vi "Server.vi"() -> ()   [LabVIEW 2019]
doc: "The myRIO Project template acquires acceleration data from the onboard accelerometer and displays the changes of acceleration values in a waveform chart."
uses:
  <vilib>/myRIO/Common/Instrument Driver Framework/myRIO v1.0/UART/vis/myRIO v1.0 Close UART.vi
  <vilib>/myRIO/Common/Instrument Driver Framework/Utilities/vis/FPGA Ref Manager.vi
  <vilib>/myRIO/Common/Instrument Driver Framework/myRIO v1.0/myRIO v1.0 Reset FPGA.vi
  <vilib>/myRIO/Common/Instrument Driver Framework/myRIO v1.0/IRQ/vis/myRIO v1.0 IRQ Info FGV.vi
  <vilib>/myRIO/Common/Instrument Driver Framework/myRIO v1.0/IRQ/vis/myRIO v1.0 Timer IRQ Info FGV.vi
  <vilib>/myRIO/Common/Instrument Driver Framework/myRIO v1.0/IRQ/vis/myRIO v1.0 ISR Agent.vi
  <vilib>/myRIO/Instrument Drivers/Utilities/vis/Reset Index.vi
  <vilib>/myRIO/Common/Instrument Driver Framework/myRIO v1.0/Resource Manager/vis/myRIO v1.0 Block Write Resource Manager.vi
  <vilib>/myRIO/Instrument Drivers/Utilities/Utilities.lvlib
panel:
  out "Waveform Chart 2":dbl(graph)
  out "Waveform Chart":dbl(graph)
  in  "Client Closed 2":string="The client VI closed the connection."
  out "OUT 2":dbl
  out "OUT":dbl
  in  "Boolean":bool
  out "output array 2":dbl[](array[numeric])
  in  "Ki 4":dbl(slide) scale=0.001..0.1
  in  "Kd 4":dbl(slide) scale=0.01..0.5
  in  "Kp 4":dbl(slide)=2.0 scale=1.0..5.0
  out "output array":dbl[](array[numeric])
  in  "Ki 3":dbl(slide) scale=0.001..0.1
  in  "Kd 3":dbl(slide) scale=0.01..0.5
  in  "Kp 3":dbl(slide)=2.0 scale=1.0..5.0
  in  "Ki 2":dbl(slide) scale=0.01..1.0
  in  "Kd 2":dbl(slide)=0.1 scale=0.001..1.0
  in  "Kp 2":dbl(slide)=3.0 scale=0.5..3.0
  in  "PWM freq [Hz] 2":dbl(slide)=250.0 scale=40.0..1000.0
  in  "Fi 2":dbl(slide) scale=-0.4..0.4
  in  "Reset Counter 2":bool
  in  "Ki 1":dbl(slide) scale=0.01..1.0
  in  "Kd 1":dbl(slide)=0.1 scale=0.001..1.0
  in  "Stop":bool
  in  "Kp 1":dbl(slide)=3.0 scale=0.5..3.0
  in  "PWM freq [Hz] 1":dbl(slide)=250.0 scale=40.0..1000.0
  in  "Fi 1":dbl(slide) scale=-0.4..0.4
  in  "Reset Counter 1":bool
  in  "Client Closed":string="The client VI closed the connection."
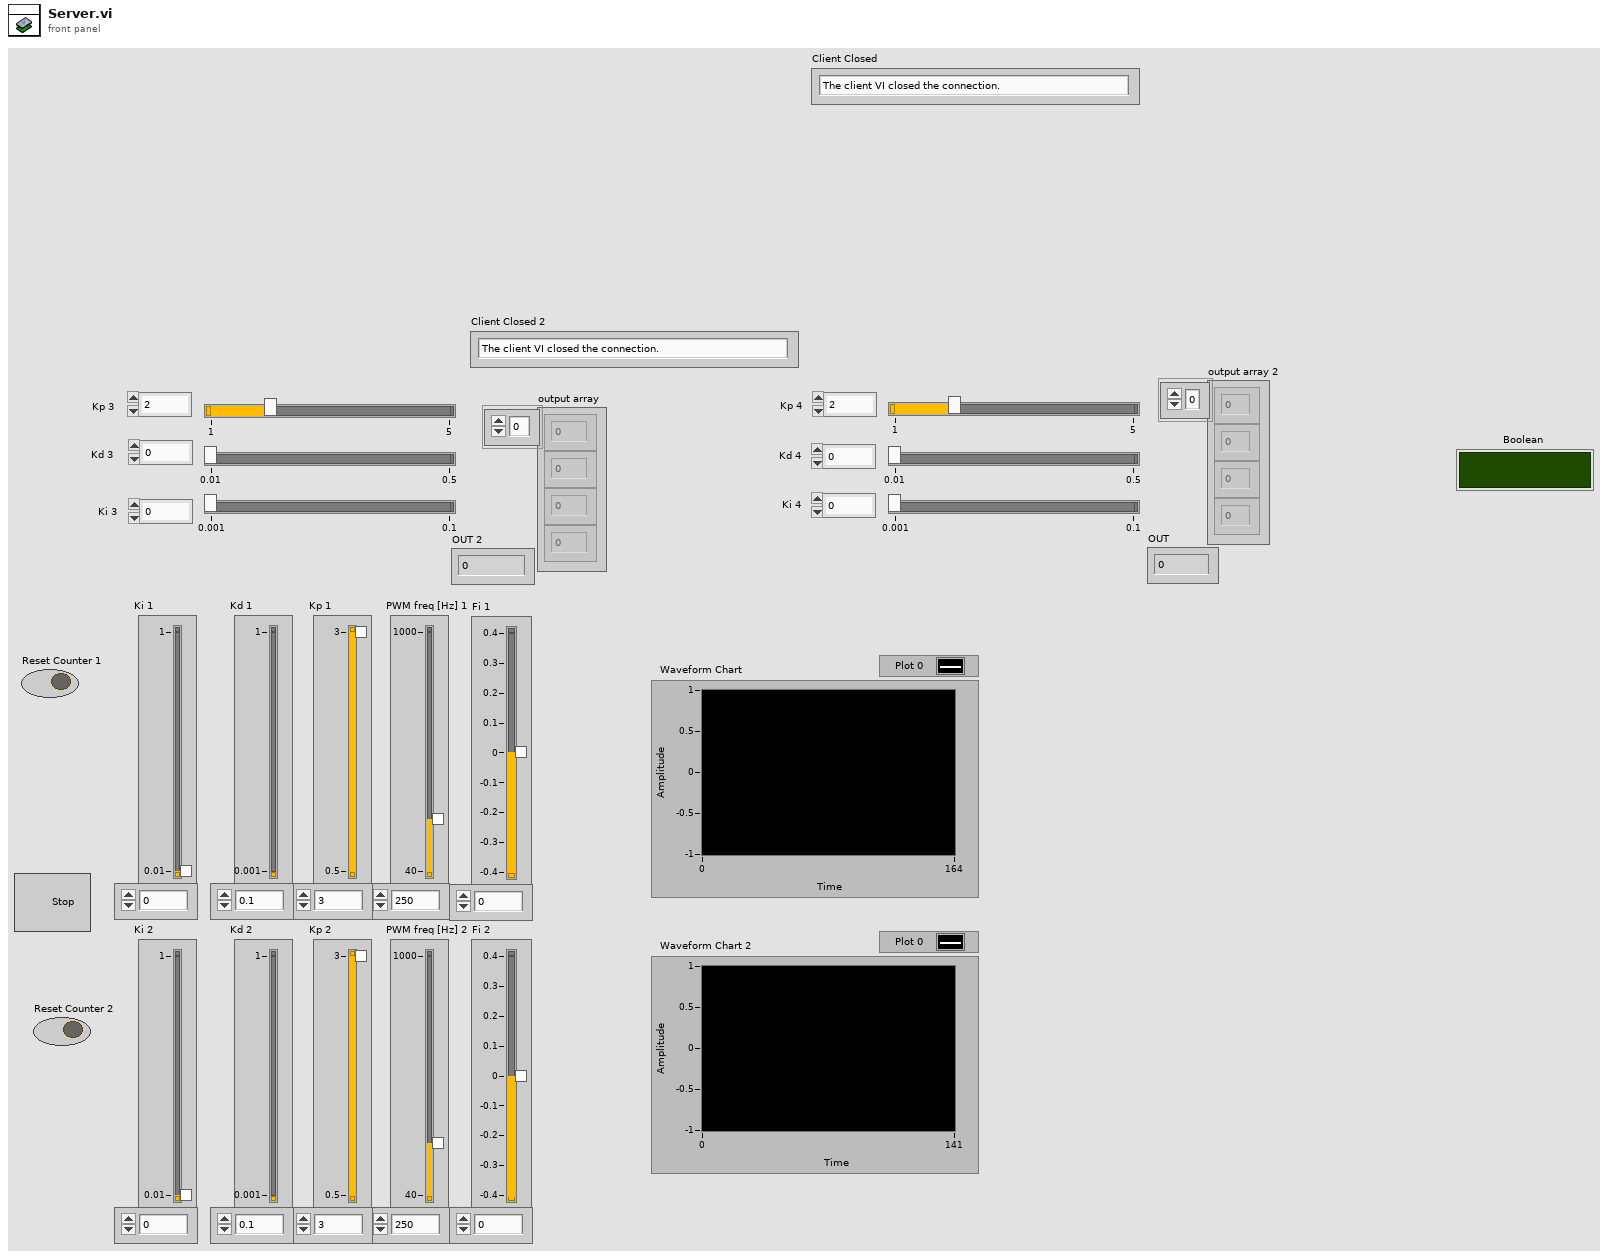
[diagram p1: front panel]
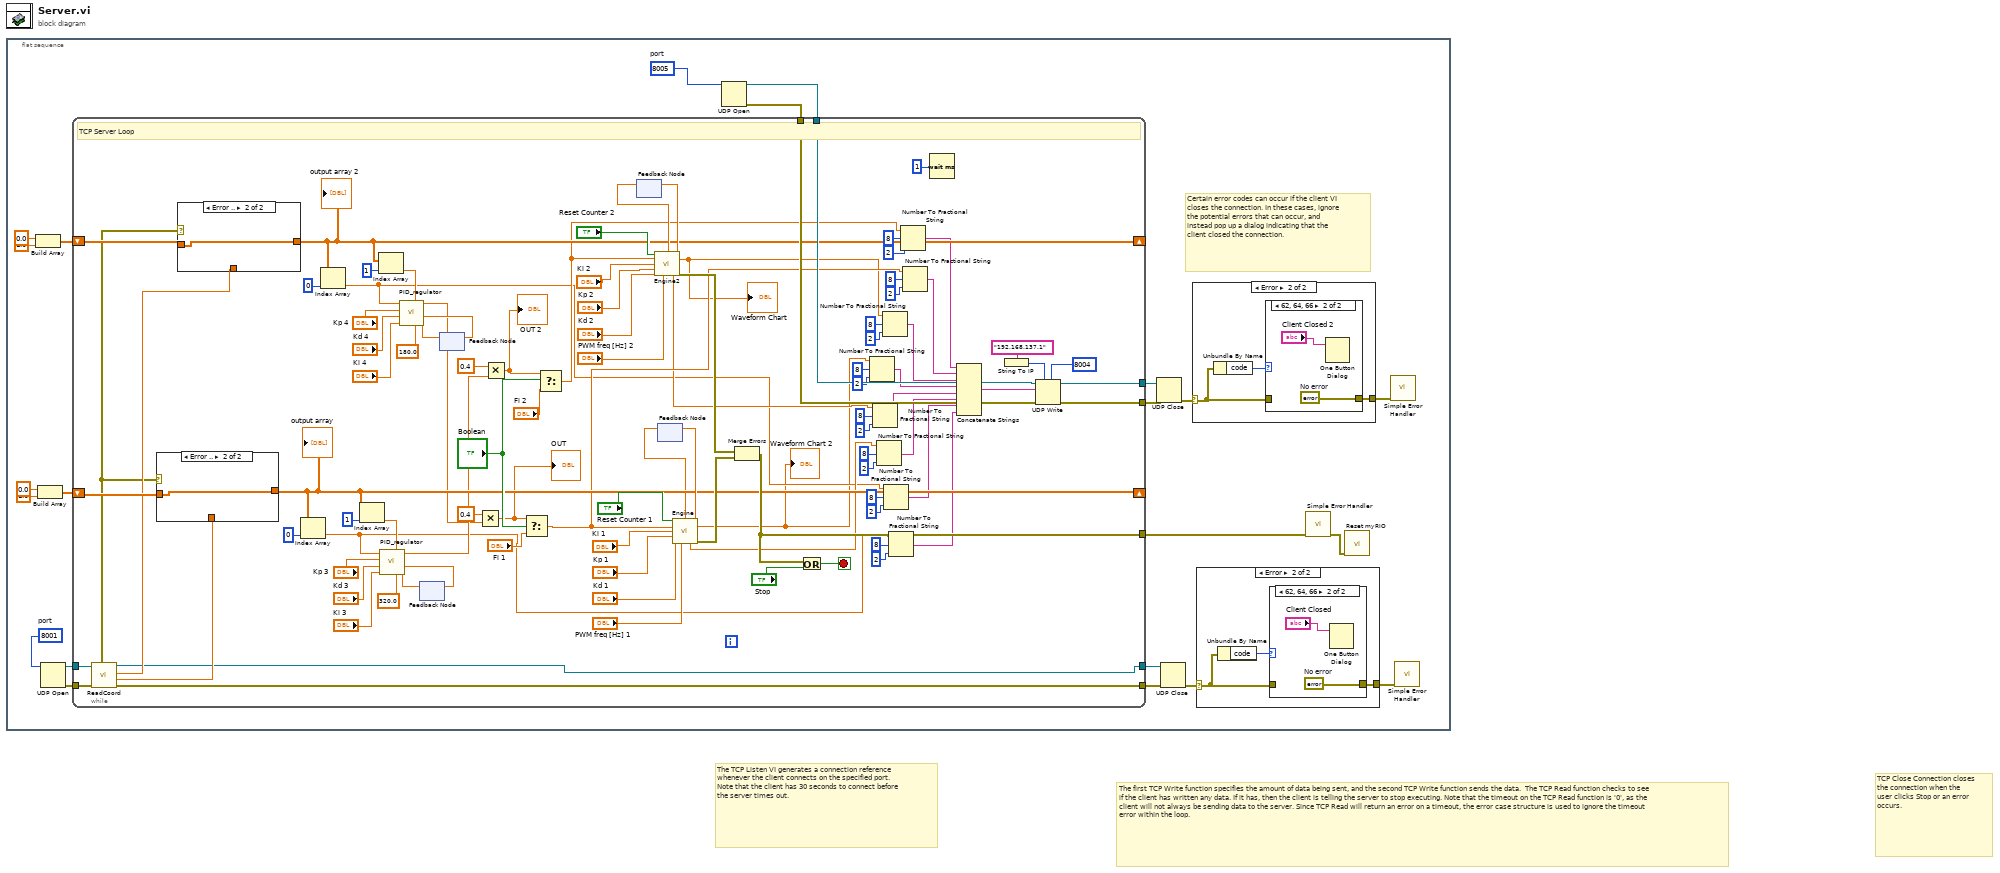
[diagram p0: block diagram]
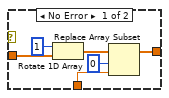
[diagram p6: hidden frame]
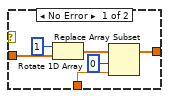
[diagram p7: hidden frame]
diagram:
  # "TCP Close Connection closes the connection when the user clicks Stop or an error occurs."
  # "The TCP Listen VI generates a connection reference whenever the client connects on the specified port. Note that the client has 30 seconds to connect before the server times out."
  # "The first TCP Write function specifies the amount of data being sent, and the second TCP Write function sends the data.  The TCP Read function checks to see if the client has written any data. If it has, then the client is telling the server to stop executing. Note that the timeout on the TCP Read function is '0', as the client will not always be sending data to the server. Since TCP Read will return an error on a timeout, the error case structure is used to ignore the timeout error within the loop."
  n1 = flat-sequence {
    frame #0 {
      w7 = u16 8005  # port
      w10 = u16 8001  # port
      # "Certain error codes can occur if the client VI closes the connection. In these cases, ignore the potential errors that can occur, and instead pop up a dialog indicating that the client closed the connection."
      n2 = Build Array(0.0 ("element"), 1.0 ("element")) -> (w11:dbl[])
      n3 = Build Array(0.0 ("element"), 1.0 ("element")) -> (w16:dbl[])
      n4 = UDP Open(11:w10) -> (port=w8:refnum<k16>, 0:w9:errorcluster)  [unwired: 4 in, 1 out]
      n5 = UDP Open(11:w7) -> (port=w6:refnum<k16>, 0:w5:errorcluster)  [unwired: 4 in, 1 out]
      n6 = while {
        tunnel: [w78] -> w21
        tunnel: [w79] -> w22
        tunnel: w8 -> [w131]
        tunnel: w9 -> [w130]
        tunnel: [w133] -> w17
        shift-right: [w91] -> _
        shift-left: w16 -> [w106]
        shift-right: [w73] -> _
        shift-left: w11 -> [w94]
        tunnel: w6 -> [w77]
        tunnel: w5 -> [w76]
        tunnel: [w75] -> w2
        tunnel: [w74] -> w1
        stop <- w134 stop-if-true
        # "TCP Server Loop"
        n7 = call "ReadCoord.vi"("error in (no error)"=w130, "connection ID"=w131) -> ("error out (no error)"=w78:errorcluster, "X"=w105:dbl, "Y"=w95:dbl, "connection ID out"=w79:refnum<k16>, "error out"=w81:errorcluster)  [unwired: 5 in]
        n8 = case shown="Error .." w81 {
          tunnel: w106 -> [w144 w148]
          tunnel: [w143 w148] -> w91
          tunnel: w105 -> [w142 _]
          frame No Error {
            n9 = Rotate 1D Array(1:w144, 2:1 ("n")) -> (0:w145:dbl[])
            n10 = Replace Array Subset(array=w145, new element=w142, index=0) -> (w143:dbl[])
          }
          frame Error {
          }
        }
        "output array" <- w91
        n11 = case shown="Error .." w81 {
          tunnel: w94 -> [w137 w141]
          tunnel: [w136 w141] -> w73
          tunnel: w95 -> [w135 _]
          frame No Error {
            n12 = Rotate 1D Array(1:w137, 2:1 ("n")) -> (0:w138:dbl[])
            n13 = Replace Array Subset(array=w138, new element=w135, index=0) -> (w136:dbl[])
          }
          frame Error {
          }
        }
        "output array 2" <- w73
        n14 = Index Array(array=w91, index=0) -> (element=w39:dbl)
        n15 = Index Array(array=w73, index=0) -> (element=w40:dbl)
        n16 = Index Array(array=w91, index=1) -> (element=w107:dbl)
        n17 = Index Array(array=w73, index=1) -> (element=w96:dbl)
        n18 = feedback #1() -> (w111:dbl)  [unwired: 1 in]
        n19 = call "PID_regulator.vi"("Integral in"=w111, "Punkt rownowagi"=320.0, "Previous IN"=w107, "Ki"="Ki 3", "Kd"="Kd 3", "Kp"="Kp 3", "IN"=w39) -> ("Integral out"=w112:dbl, "OUT"=w87:dbl)  [unwired: 3 in]
        n20 = feedback-in #1(w112) -> ()
        n21 = feedback #2() -> (w100:dbl)  [unwired: 1 in]
        n22 = call "PID_regulator.vi"("Integral in"=w100, "Punkt rownowagi"=180.0, "Previous IN"=w96, "Ki"="Ki 4", "Kd"="Kd 4", "Kp"="Kp 4", "IN"=w40) -> ("Integral out"=w101:dbl, "OUT"=w85:dbl)  [unwired: 3 in]
        n23 = feedback-in #2(w101) -> ()
        n24 = Multiply(x=0.4, y=w85) -> (x*y=w82:dbl)
        "OUT" <- w82
        n25 = Multiply(x=0.4, y=w87) -> (x*y=w83:dbl)
        "OUT 2" <- w83
        n26 = Select(t=w82, s="Boolean", f="Fi 1") -> (s? t:f=w43:dbl)
        n27 = Select(t=w83, s="Boolean", f="Fi 2") -> (s? t:f=w44:dbl)
        n28 = feedback #3() -> (w89:dbl)  [unwired: 1 in]
        n29 = call "Engine2.vi"("Reset Counter"="Reset Counter 2", "Integral in"=w89, "Fi"=w44, "Ki"="Ki 2", "Kp"="Kp 2", "Kd"="Kd 2", "PWM freq [Hz]"="PWM freq [Hz] 2") -> ("Integral out"=w123:dbl, "fi"=w38:dbl, "PWM"=w42:dbl, "error out"=w124:errorcluster)  [unwired: 3 in, 2 out]
        "Waveform Chart" <- w38
        n30 = feedback-in #3(w123) -> ()
        n31 = feedback #4() -> (w88:dbl)  [unwired: 1 in]
        n32 = call "Engine.vi"("Reset Counter"="Reset Counter 1", "Integral in"=w88, "Fi"=w43, "Ki"="Ki 1", "Kp"="Kp 1", "Kd"="Kd 1", "PWM freq [Hz] in"="PWM freq [Hz] 1") -> ("Integral out"=w121:dbl, "fi"=w37:dbl, "pwm"=w41:dbl, "error out"=w122:errorcluster)  [unwired: 2 in, 3 out]
        "Waveform Chart 2" <- w37
        n33 = feedback-in #4(w121) -> ()
        n34 = Merge Errors(w124, w122) -> (w133:errorcluster)
        n35 = Or(x=w133, y="Stop") -> (x .or. y?=w134:bool)
        n36 = Number To Fractional String(number=w37, width (-)=i16 8, precision (6)=i16 2) -> (F-format string=w57:string)  [unwired: 1 in]
        n37 = Number To Fractional String(number=w42, width (-)=i16 8, precision (6)=i16 2) -> (F-format string=w54:string)  [unwired: 1 in]
        n38 = Number To Fractional String(number=w41, width (-)=i16 8, precision (6)=i16 2) -> (F-format string=w51:string)  [unwired: 1 in]
        n39 = Number To Fractional String(number=w38, width (-)=i16 8, precision (6)=i16 2) -> (F-format string=w60:string)  [unwired: 1 in]
        n40 = Number To Fractional String(number=w40, width (-)=i16 8, precision (6)=i16 2) -> (F-format string=w48:string)  [unwired: 1 in]
        n41 = Number To Fractional String(number=w39, width (-)=i16 8, precision (6)=i16 2) -> (F-format string=w45:string)  [unwired: 1 in]
        n42 = Number To Fractional String(number=w44, width (-)=i16 8, precision (6)=i16 2) -> (F-format string=w66:string)  [unwired: 1 in]
        n43 = Number To Fractional String(number=w43, width (-)=i16 8, precision (6)=i16 2) -> (F-format string=w63:string)  [unwired: 1 in]
        n44 = Wait (ms)(milliseconds to wait=u32 1) -> ()  [unwired: 1 out]
        n45 = Concatenate Strings(w66, w63, w60, w57, w54, w51, w48, w45) -> (w67:string)
        n46 = String To IP(1:"192.168.137.1" ("name")) -> (0:w72:u32)
        n47 = UDP Write(address=w72, port or service name=u16 8004, connection ID=w77, data in=w67, 8:w76) -> (error out=w74:errorcluster, 3:w75:refnum<k16>)  [unwired: 1 in]
      }
      n48 = UDP Close(connection ID=w2, 8:w1) -> (error out=w4:errorcluster)  [unwired: 1 out]
      n49 = UDP Close(connection ID=w22, 8:w21) -> (error out=w20:errorcluster)  [unwired: 1 out]
      n50 = case shown="Error" w4 {
        selector: w4 -> [w23 w25]
        tunnel: [w23 w24] -> w3
        frame No Error {
        }
        frame Error {
          n51 = Unbundle By Name(w25) -> ("code"=w26:i32)
          n52 = case shown="62, 64, 66" w26 {
            tunnel: w25 -> [w27 _]
            tunnel: [w27 w29] -> w24
            frame Default {
            }
            frame 62, 64, 66 {
              w29 = errorcluster {"status"=FALSE, "code"=0, "source"=""}  # No error
              n53 = One Button Dialog(message="Client Closed 2") -> ()  [unwired: 1 in, 1 out]
            }
          }
        }
      }
      n54 = case shown="Error" w20 {
        selector: w20 -> [w30 w32]
        tunnel: [w30 w31] -> w19
        frame No Error {
        }
        frame Error {
          n55 = Unbundle By Name(w32) -> ("code"=w33:i32)
          n56 = case shown="62, 64, 66" w33 {
            tunnel: w32 -> [w34 _]
            tunnel: [w34 w36] -> w31
            frame Default {
            }
            frame 62, 64, 66 {
              w36 = errorcluster {"status"=FALSE, "code"=0, "source"=""}  # No error
              n57 = One Button Dialog(message="Client Closed") -> ()  [unwired: 1 in, 1 out]
            }
          }
        }
      }
      n58 = call <vilib>:"Simple Error Handler.vi"("error in (no error)"=w17) -> ("error out"=w18:errorcluster)  [unwired: 4 in, 4 out]
      n59 = call <vilib>:"Reset myRIO.vi"("error in (no error)"=w18) -> ()  [unwired: 10 in, 1 out]
      n60 = call <vilib>:"Simple Error Handler.vi"("error in (no error)"=w3) -> ()  [unwired: 1 in, 8 out]
      n61 = call <vilib>:"Simple Error Handler.vi"("error in (no error)"=w19) -> ()  [unwired: 1 in, 8 out]
    }
  }
